vi "LAOnChunk.vi"(8 "Error In":errorcluster, 11 "LiteAgent In":T2) -> (0 "Error Out":errorcluster, 1 "AgentMessageChunk":T1, 2 "SessionId":string, 3 "LiteAgent Out":T2)   [LabVIEW 2017, in "LiteAgentSDK.lvlib"]
uses:
  LiteAgentSDK.lvlib
  C:/Users/Jan/Projects/LiteAgentSDK-LabVIEW/Source/Bin/LiteAgentSDK.LabVIEW.dll
  Bin/LiteAgentSDK.LabVIEW.dll
  <vilib>/LVH/i3 JSON/JSON Parsing/Get Object Parameter Files/Get Object Parameter - String.vi
  <vilib>/LVH/i3 JSON/JSON Parsing/Get Object Parameter Files/Get Object Parameter - Object.vi
  <vilib>/LVH/i3 JSON/i3-json.lvlib
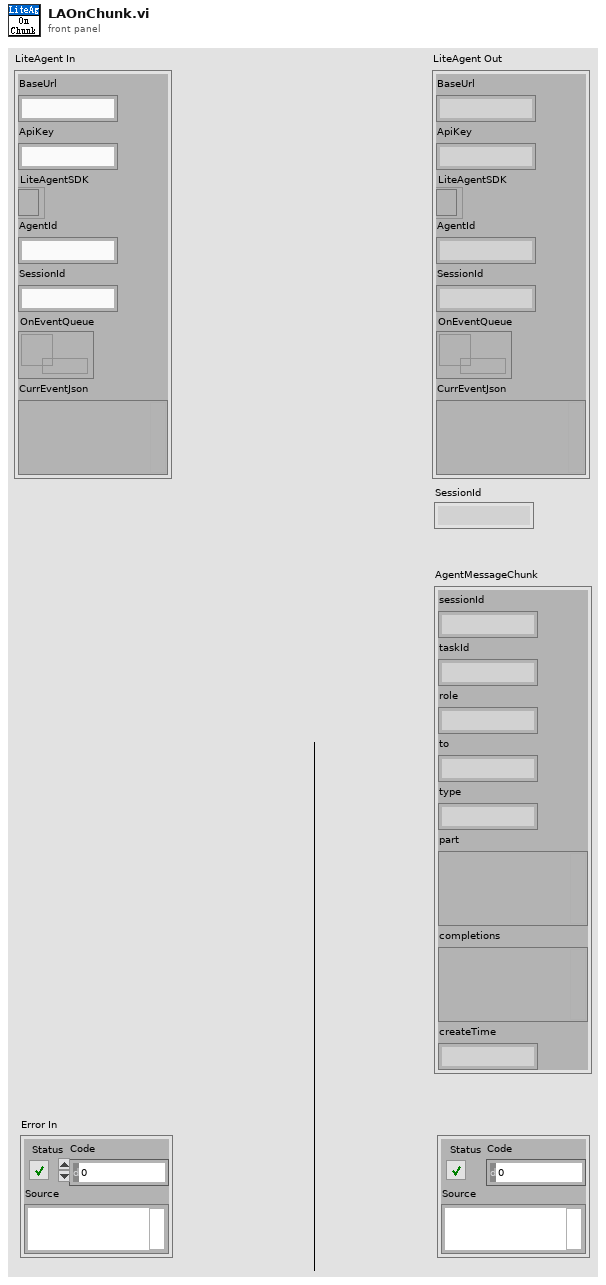
[diagram p1: front panel]
types:
  T1 = cluster{"sessionId":string, "taskId":string, "role":string, "to":string, "type":string, "part":variant, "completions":variant, "createTime":string}
  T2 = cluster{"BaseUrl":string, "ApiKey":string, "LiteAgentSDK":refnum<k24>, "AgentId":string, "SessionId":string, "OnEventQueue":refnum<queue>, "CurrEventJson":variant}
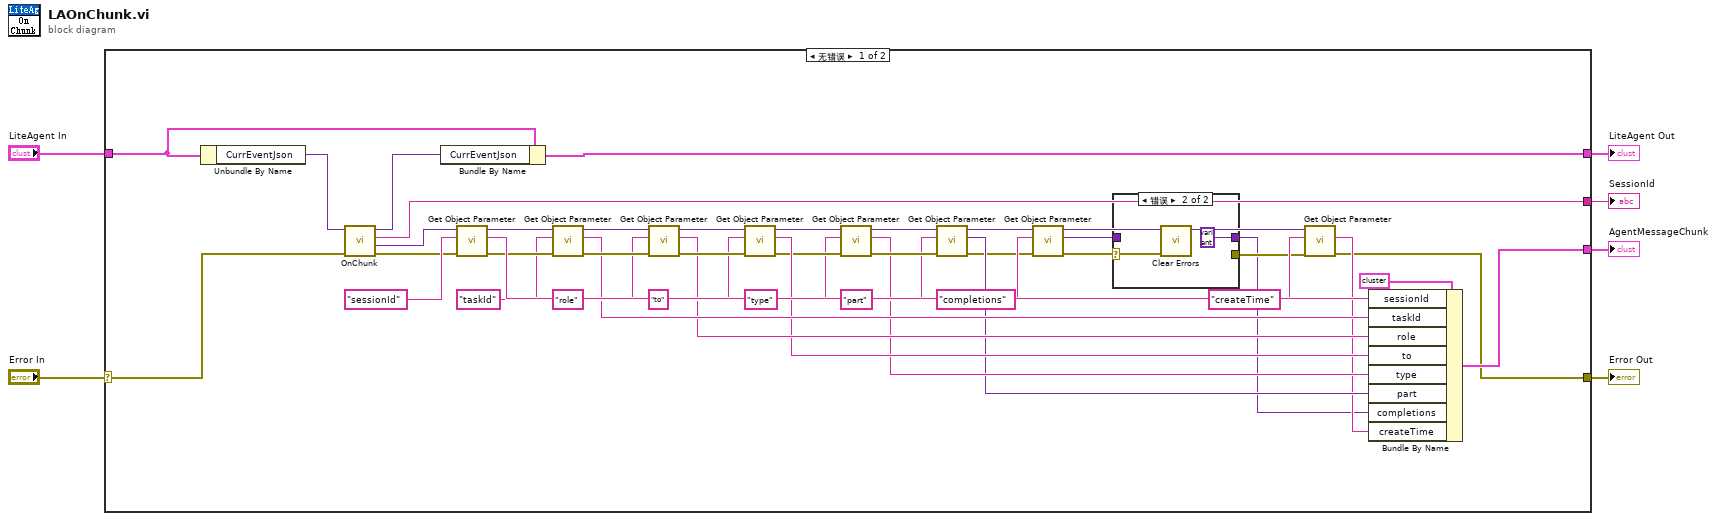
[diagram p0: block diagram]
diagram:
  n1 = case shown="无错误" "Error In" {
    selector: "Error In" -> [w49 w55]
    tunnel: [w12 w55] -> w5
    tunnel: "LiteAgent In" -> [w47 w54]
    tunnel: [w45 w54] -> w3
    tunnel: [w13 _] -> w2
    tunnel: [w14 _] -> w1
    frame No Error {
      n2 = Unbundle By Name(w47) -> ("CurrEventJson"=w48:variant)
      n3 = call "OnChunk.vi"("Error In"=w49, "JSON Tree In"=w48) -> ("Error Out"=w17:errorcluster, "Payload"=w16:variant, "SessionId"=w13:string, "JSON Tree Out"=w46:variant)  [unwired: 6 in]
      n4 = Bundle By Name(cluster=w47, "CurrEventJson"=w46) -> (w45:T2)
      n5 = call-poly <vilib>:"Get Object Parameter.vi"("error in (no error)"=w17, "Parameter Name"="sessionId", "JSON Tree In (JSON Object)"=w16) -> ("error out"=w41:errorcluster, "String Value"=w43:string, "JSON Tree Out Passthrough"=w42:variant)  [unwired: 5 in, 1 out]
      n6 = call-poly <vilib>:"Get Object Parameter.vi"("error in (no error)"=w41, "Parameter Name"="taskId", "JSON Tree In (JSON Object)"=w42) -> ("error out"=w38:errorcluster, "String Value"=w33:string, "JSON Tree Out Passthrough"=w40:variant)  [unwired: 5 in, 1 out]
      n7 = call-poly <vilib>:"Get Object Parameter.vi"("error in (no error)"=w38, "Parameter Name"="role", "JSON Tree In (JSON Object)"=w40) -> ("error out"=w37:errorcluster, "String Value"=w32:string, "JSON Tree Out Passthrough"=w39:variant)  [unwired: 5 in, 1 out]
      n8 = call-poly <vilib>:"Get Object Parameter.vi"("error in (no error)"=w37, "Parameter Name"="to", "JSON Tree In (JSON Object)"=w39) -> ("error out"=w26:errorcluster, "String Value"=w31:string, "JSON Tree Out Passthrough"=w30:variant)  [unwired: 5 in, 1 out]
      n9 = call-poly <vilib>:"Get Object Parameter.vi"("error in (no error)"=w26, "Parameter Name"="type", "JSON Tree In (JSON Object)"=w30) -> ("error out"=w25:errorcluster, "String Value"=w20:string, "JSON Tree Out Passthrough"=w29:variant)  [unwired: 5 in, 1 out]
      n10 = call-poly <vilib>:"Get Object Parameter.vi"("error in (no error)"=w25, "Parameter Name"="part", "JSON Tree In (JSON Object)"=w29) -> ("error out"=w11:errorcluster, "JSON Object"=w19:variant, "JSON Tree Out Passthrough"=w28:variant)  [unwired: 5 in, 1 out]
      n11 = call-poly <vilib>:"Get Object Parameter.vi"("error in (no error)"=w11, "Parameter Name"="completions", "JSON Tree In (JSON Object)"=w28) -> ("error out"=w10:errorcluster, "JSON Object"=w8:variant, "JSON Tree Out Passthrough"=w27:variant)  [unwired: 5 in, 1 out]
      n12 = case shown="错误" w10 {
        selector: w10 -> [w51 w53]
        tunnel: [w51 _] -> w9
        tunnel: w8 -> [w50 _]
        tunnel: [w50 variant ("JSON Object")] -> w7
        frame No Error {
        }
        frame Error {
          n13 = call <vilib>:"Clear Errors.vi"("error in (no error)"=w53) -> ()  [unwired: 5 in, 2 out]
        }
      }
      n14 = call-poly <vilib>:"Get Object Parameter.vi"("error in (no error)"=w9, "Parameter Name"="createTime", "JSON Tree In (JSON Object)"=w27) -> ("error out"=w12:errorcluster, "String Value"=w18:string)  [unwired: 5 in, 2 out]
      n15 = Bundle By Name(cluster=T1 {"sessionId"="", "taskId"="", "role"="", "to"="", "type"="", "part"=variant, "completions"=variant, "createTime"=""} ("AgentMessageChunk"), "sessionId"=w43, "taskId"=w33, "role"=w32, "to"=w31, "type"=w20, "part"=w19, "completions"=w7, "createTime"=w18) -> (w14:T1)
    }
    frame Error {
    }
  }
  "Error Out" <- w5
  "LiteAgent Out" <- w3
  "SessionId" <- w2
  "AgentMessageChunk" <- w1
